vi "RSB_ext.vi"(3 "Q old":bool[](array[boolean]), 4 "R":bool[](array[boolean]), 5 "S":bool[](array[boolean])) -> (1 "~Q":bool[](array[boolean]), 2 "Q":bool[](array[boolean]))   [LabVIEW 2019, in "Triggers.lvlib"]
uses:
  Triggers.lvlib
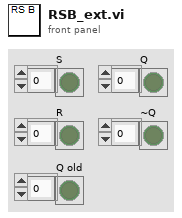
[diagram p1: front panel]
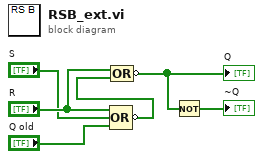
[diagram p0: block diagram]
diagram:
  n1 = Compound Arithmetic op=OR("R", "S", "Q old") -> (invert w5:bool[])
  n2 = Compound Arithmetic op=OR("R", w5) -> (invert w3:bool[])
  "Q" <- w3
  n3 = Not(x=w3) -> (.not. x?=→"~Q":bool[])
